vi "Generate Test Parameter Globals_1.0.0.vi"(9 "Column Headers In":string[](array[string]), 11 "file path (dialog if empty)":path=path "C:/IdtATE/Infrastructure/Test Parameters.tmp") -> (1 "Test Parameters":string[][](array[string]), 3 "# of iterations":i32)   [LabVIEW 2018]
uses:
  <vilib>/Utility/file.llb/Read From Spreadsheet File (string).vi
  Test Parameter Globals_1.0.0.vi
panel:
  out "Column Headers Global":string[](array[string])
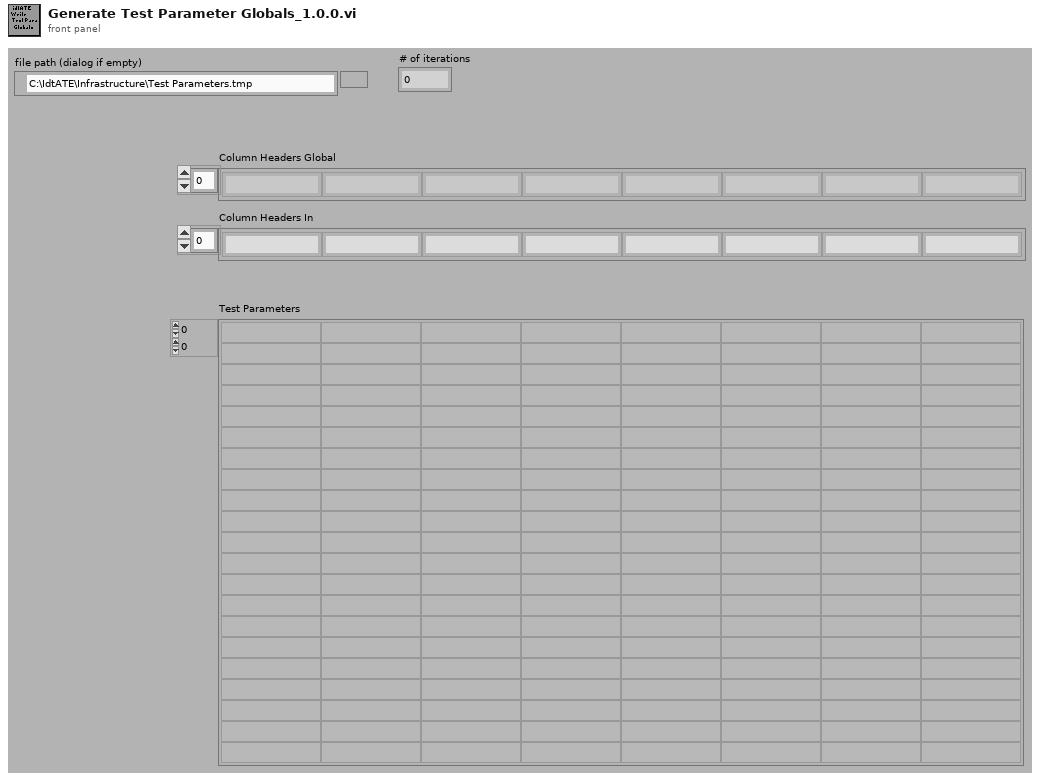
[diagram p1: front panel]
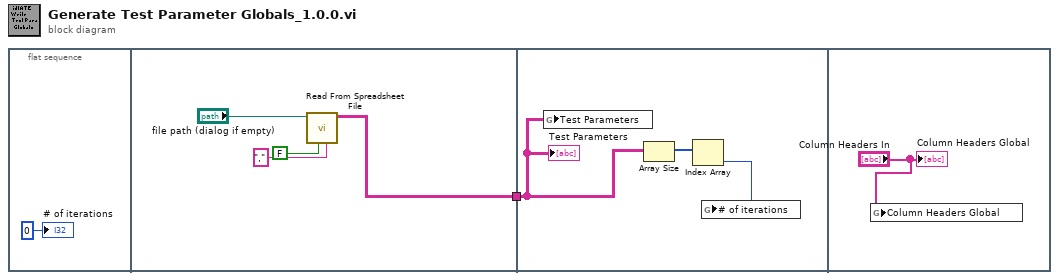
[diagram p0: block diagram]
diagram:
  n1 = flat-sequence {
    tunnel: [w3] -> w1
    tunnel: w1 -> [w9]
    frame #0 {
      "# of iterations" <- 0 ("# of iterations")
    }
    frame #1 {
      n2 = call-poly <vilib>:"Read From Spreadsheet File.vi"("delimiter (\\t)"="," ("delimiter (\\t)"), "transpose (no:F)"=FALSE, "file path (dialog if empty)"="file path (dialog if empty)") -> ("all rows"=w3:string[][])  [unwired: 4 in, 4 out]
    }
    frame #2 {
      n3 = global write "Test Parameter Globals_1.0.0.vi" "Test Parameters"(w9) -> ()
      n4 = Array Size(array=w9) -> (size(s)=w8:i32[])
      n5 = Index Array(array=w8) -> (element=w7:i32)  [unwired: 1 in]
      n6 = global write "Test Parameter Globals_1.0.0.vi" "# of iterations"(w7) -> ()
      "Test Parameters" <- w9
    }
    frame #3 {
      n7 = global write "Test Parameter Globals_1.0.0.vi" "Column Headers Global"("Column Headers In") -> ()
      "Column Headers Global" <- "Column Headers In"
    }
  }
